vi "example.vi"() -> ()   [LabVIEW 2018]
panel:
  in  "Array":dbl[](array[numeric])
  in  "stop":bool
  in  "list1":dbl[](array[numeric])
  out "new list":i32[](array[numeric])
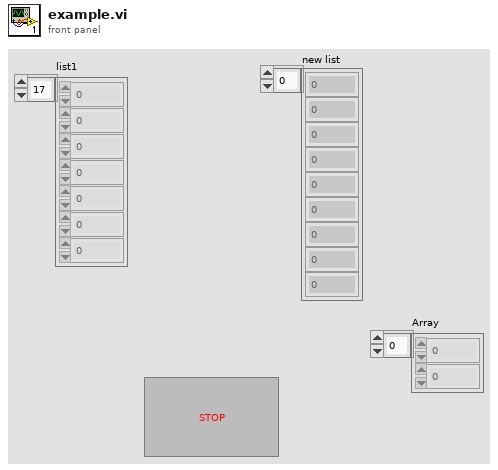
[diagram p1: front panel]
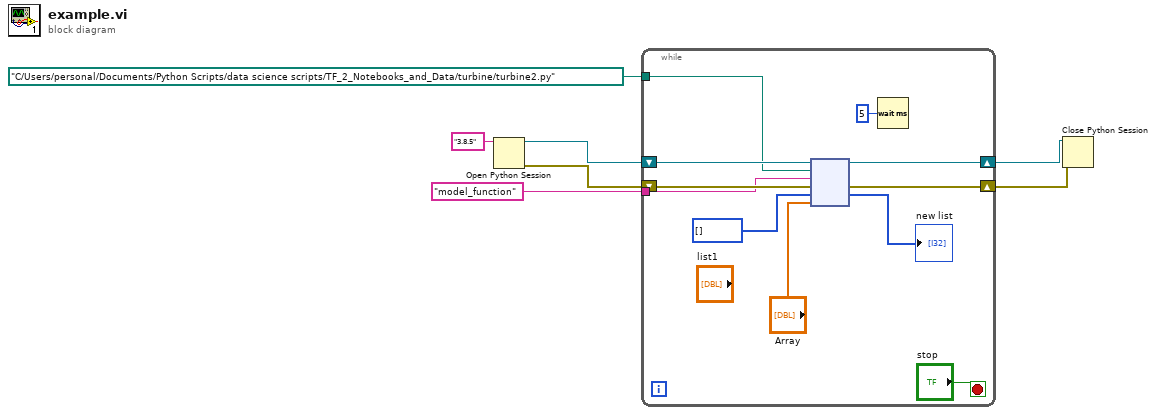
[diagram p0: block diagram]
diagram:
  n1 = Open Python Session(python version="3.8.5" ("Python version")) -> (session out=w7:refnum<k35>, error out=w6:errorcluster)  [unwired: 2 in]
  n2 = while {
    tunnel: path "C:/Users/personal/Documents/Python Scripts/data science scripts/TF_2_Notebooks_and_Data/turbine/turbine2.py" ("module path") -> [w14]
    tunnel: "model_function" ("function name") -> [w13]
    shift-right: [w16] -> w5
    shift-left: w7 -> [w18]
    shift-right: [w15] -> w4
    shift-left: w6 -> [w17]
    stop <- "stop" stop-if-true
    n3 = node(w18, w14, w13, w17, i32[] [], "Array") -> (w16:refnum<k35>, w15:errorcluster, →"new list":i32[])  [unwired: 1 in, 2 out]
    n4 = Wait (ms)(milliseconds to wait=u32 5) -> ()  [unwired: 1 out]
  }
  n5 = Close Python Session(session in=w5, error in=w4) -> ()  [unwired: 1 out]
